vi "Set Current Path for Visualization.vi"(11 "Path":cluster{dbl, "interpolation value":dbl}[](array[cluster])) -> ()   [LabVIEW 2017, in "Pure Pursuit.lvlib"]
uses:
  Current Path.vi
  Pure Pursuit.lvlib
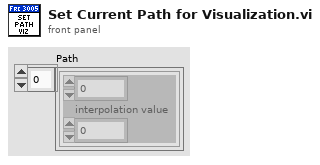
[diagram p1: front panel]
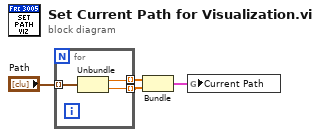
[diagram p0: block diagram]
diagram:
  n1 = for {
    tunnel: [w7] -> _ mode=indexing
    tunnel: "Path" -> [w7] mode=indexing
    tunnel: [w6] -> w3 mode=indexing
    tunnel: [w5] -> w2 mode=indexing
    n2 = Unbundle(w7) -> (w5:dbl, "interpolation value"=w6:dbl)
  }
  n3 = Bundle(w2, w3) -> (w1:cluster{dbl[], dbl[]})  [unwired: 1 in]
  n4 = global write "Current Path.vi" "Current Path"(w1) -> ()
